vi "A3(SubVI).vi"(8 "error in (no error)":errorcluster) -> (0 "error out":errorcluster, 1 "A(ZN)":dbl[](array[numeric]), 2 "A(KN)":dbl[](array[numeric]), 3 "A(TS)":dbl[](array[numeric]), 5 "Absorbancs Graph":cluster{dbl[], dbl[]}[](graph))   [LabVIEW 2019]
uses:
  Global.vi
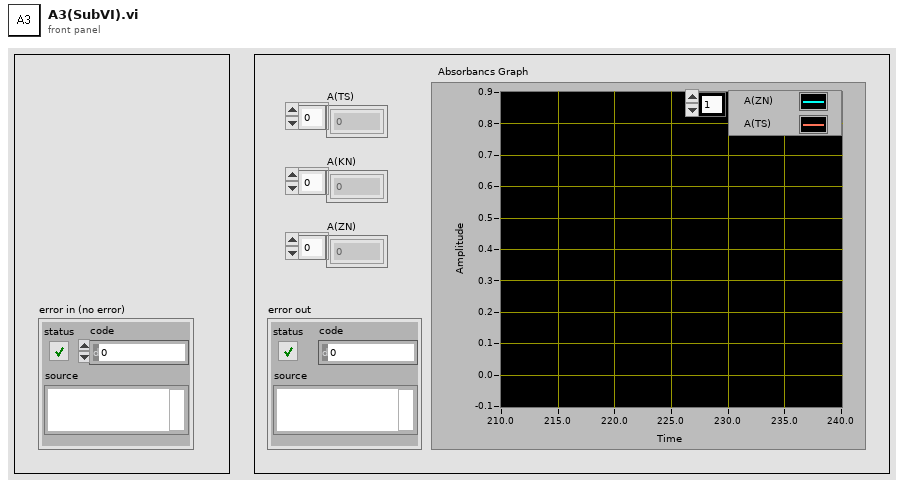
[diagram p1: front panel]
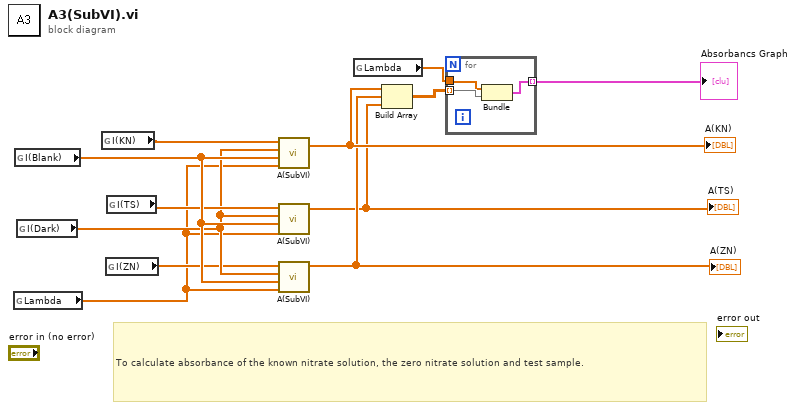
[diagram p0: block diagram]
diagram:
  # "To calculate absorbance of the known nitrate solution, the zero nitrate solution and test sample."
  n1 = global read "Global.vi" "Lambda"() -> (w3:dbl[])
  n2 = global read "Global.vi" "I(Blank)"() -> (w7:dbl[])
  n3 = global read "Global.vi" "I(Dark)"() -> (w5:dbl[])
  n4 = global read "Global.vi" "I(KN)"() -> (w8:dbl[])
  n5 = global read "Global.vi" "I(ZN)"() -> (w4:dbl[])
  n6 = global read "Global.vi" "I(TS)"() -> (w6:dbl[])
  n7 = call "A(SubVI).vi"("Lambda"=w3, "I(blank)"=w7, "I(dark)"=w5, "I"=w8) -> ("Aout"=w11:dbl[])  [unwired: 7 in]
  "A(KN)" <- w11
  n8 = call "A(SubVI).vi"("Lambda"=w3, "I(blank)"=w7, "I(dark)"=w5, "I"=w6) -> ("Aout"=w1:dbl[])  [unwired: 7 in]
  "A(TS)" <- w1
  n9 = call "A(SubVI).vi"("Lambda"=w3, "I(blank)"=w7, "I(dark)"=w5, "I"=w4) -> ("Aout"=w2:dbl[])  [unwired: 7 in]
  "A(ZN)" <- w2
  n10 = global read "Global.vi" "Lambda"() -> (w12:dbl[])
  n11 = Build Array(w11, w2, w1) -> (w9:dbl[][])
  n12 = for {
    tunnel: w9 -> [w15] mode=indexing
    tunnel: [w14] -> w10 mode=indexing
    tunnel: w12 -> [w13]
    n13 = Bundle("Lambda"=w13, w15) -> (w14:cluster{"Lambda":dbl[], dbl[]})  [unwired: 1 in]
  }
  "Absorbancs Graph" <- w10
